vi "Receive.vi"(8 "error in (no error)":errorcluster, 9 "timeout in ms (-1)":i32=-1, 11 "JQMHStartup in":refnum<class "JQMHStartup.lvclass">) -> (0 "error out":errorcluster, 1 "Data":variant, 2 "Command":string, 3 "JQMHStartup out":refnum<class "JQMHStartup.lvclass">, 4 "timed out?":bool)   [LabVIEW 2024, in "JQMHStartup.lvclass"]
uses:
  JQMHStartup.lvclass
  JQMHStartup.lvclass/JQMHStartup.ctl
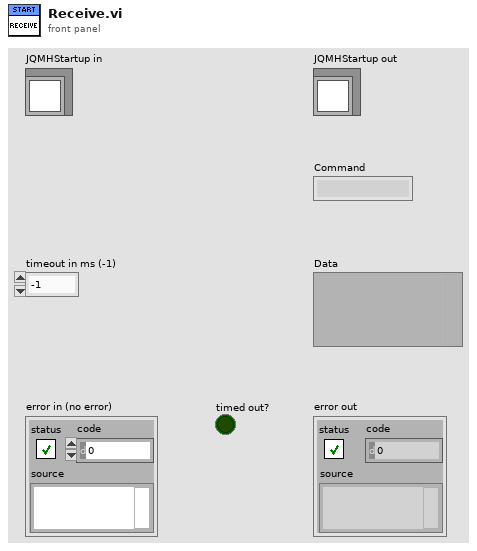
[diagram p1: front panel]
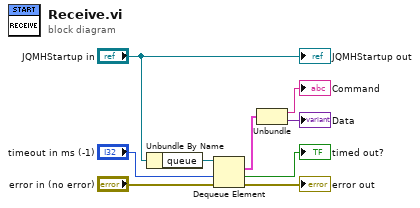
[diagram p0: block diagram]
diagram:
  n1 = Unbundle By Name("JQMHStartup in") -> ("queue"=w8:refnum<queue>)
  n2 = Dequeue Element(queue=w8, timeout in ms (-1)="timeout in ms (-1)", error in (no error)="error in (no error)") -> (element=w3:cluster{string, variant}, timed out?=→"timed out?":bool, error out=→"error out":errorcluster)  [unwired: 1 out]
  n3 = Unbundle(w3) -> (→"Command":string, →"Data":variant)
  "JQMHStartup out" <- "JQMHStartup in"
